vi "Start Measurement.vi"(8 "error in (no error)":errorcluster, 9 "Device Names":string[](array[string]), 10 "Measurement Name":string, 11 "Mag Lab Measure Controller in":refnum<class "Mag Lab Measure Controller.lvclass">) -> (0 "error out":errorcluster, 3 "Mag Lab Measure Controller out":refnum<class "Mag Lab Measure Controller.lvclass">)   [LabVIEW 2015, in "Mag Lab Measure Controller.lvclass"]
uses:
  Mag Lab Measure Controller.lvclass
  Mag Lab Root/Mag Lab Root.lvclass/Mag Lab Root.ctl
  <vilib>/ActorFramework/Actor/Actor.lvclass/Actor.ctl
  <vilib>/ActorFramework/Message Enqueuer/Message Enqueuer.lvclass/Message Enqueuer.ctl
  Mag Lab Measure Controller Messages/Log Status Update Msg/Log Status Update Msg.lvclass/Log Status Update Msg.ctl
  Mag Lab Root Messages/Initialize Msg/Initialize Msg.lvclass/Initialize Msg.ctl
  <vilib>/ActorFramework/Message Enqueuer/Init from Existing Queue.vi
  <vilib>/ActorFramework/Message Enqueuer/Enqueue.vi
  <vilib>/ActorFramework/Message Priority Queue/Priority Enqueue.vi
  <vilib>/ActorFramework/Message Enqueuer/Message Enqueuer.lvclass
  Mag Lab Measure Controller Messages/Log Status Update Msg/Log Status Update Msg.lvclass
  Mag Lab Root Messages/Initialize Msg/Initialize Msg.lvclass
  <vilib>/ActorFramework/Actor/Actor.lvclass
  Mag Lab Error Handler/Mag Lab Error Handler.lvclass
  Mag Lab Measure Base/Mag Lab Measure Base.lvclass
  Mag Lab Root/Mag Lab Root.lvclass
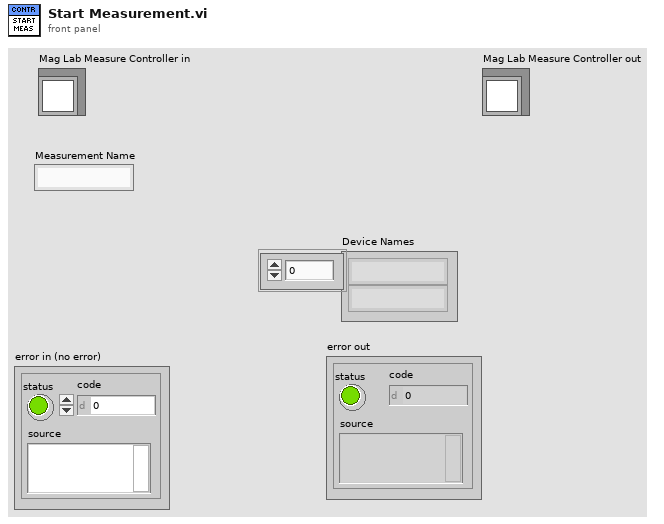
[diagram p1: front panel]
types:
  T1 = cluster{"Measurement Name":string, "Device Names":string[]}
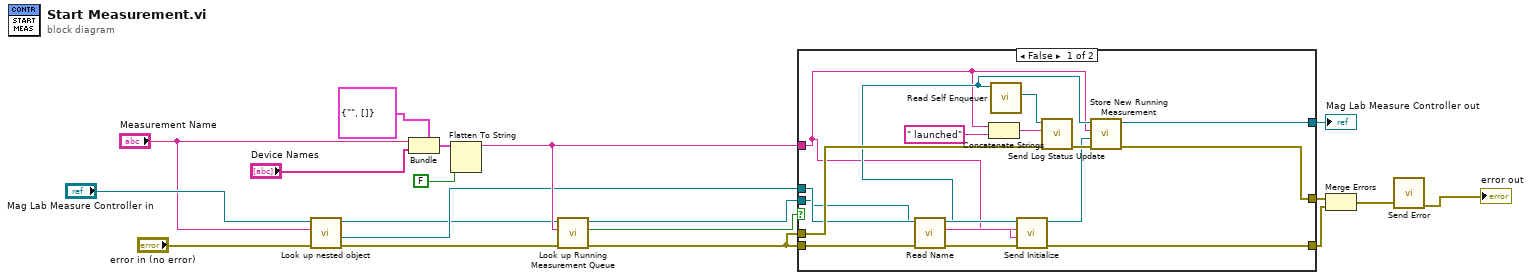
[diagram p0: block diagram]
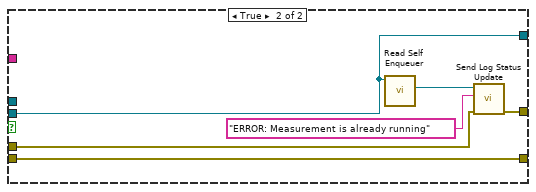
[diagram p2: hidden frame]
diagram:
  n1 = call "Look up nested object.vi"("error in (no error)"="error in (no error)", "Object name"="Measurement Name", "Mag Lab Measure Base in"="Mag Lab Measure Controller in") -> ("error out"=w2:errorcluster, "Object Queue"=w6:refnum<class "Message Enqueuer.lvclass">, "Mag Lab Measure Base out"=w5:refnum<class "Mag Lab Measure Controller.lvclass">)  [unwired: 5 in, 1 out]
  n2 = Bundle(cluster=T1 {"Measurement Name"="", "Device Names"=[]} ("output cluster"), "Measurement Name"="Measurement Name", "Device Names"="Device Names") -> (w18:T1)
  n3 = Flatten To String(anything=w18, prepend array or string size? (T)=FALSE) -> (data string=w14:string)  [unwired: 2 in, 2 out]
  n4 = call "Look up Running Measurement Queue .vi"("error in (no error)"=w2, "Measurement Name.Harware()"=w14, "Mag Lab Measure Controller in"=w5) -> ("error out"=w11:errorcluster, "Found?"=w13:bool, "Mag Lab Measure Controller out"=w12:refnum<class "Mag Lab Measure Controller.lvclass">)  [unwired: 4 in, 1 out]
  n5 = case shown="False" w13 {
    tunnel: [w35 w41] -> w10
    tunnel: w6 -> [w28 _]
    tunnel: w14 -> [w20 _]
    tunnel: w12 -> [w25 w41]
    tunnel: w11 -> [w30 w39]
    tunnel: [w33 w38] -> w15
    tunnel: w11 -> [w22 w40]
    tunnel: [w26 w40] -> w16
    frame False {
      n6 = call "Read Name.vi"("error in (no error)"=w22, "Mag Lab Root in"=w25) -> ("error out"=w23:errorcluster, "Name"=w21:string, "Mag Lab Root out"=w24:refnum<class "Mag Lab Measure Controller.lvclass">)  [unwired: 7 in]
      n7 = Concatenate Strings(w20, " launched" ("string")) -> (w31:string)
      n8 = call <vilib>:"Read Self Enqueuer.vi"("Actor"=w24) -> ("Self Enqueuer"=w32:refnum<class "Message Enqueuer.lvclass">)  [unwired: 10 in]
      n9 = call "Send Initialize.vi"("error in (no error)"=w23, "Requestor"=w21, "Requestee"=w20, "Message Enqueuer"=w28) -> ("error out"=w26:errorcluster, "Message Enqueuer out"=w27:refnum<class "Message Enqueuer.lvclass">)  [unwired: 6 in]
      n10 = call "Send Log Status Update.vi"("error in (no error)"=w30, "Status"=w31, "Message Enqueuer"=w32) -> ("error out"=w29:errorcluster)  [unwired: 7 in, 1 out]
      n11 = call "Store New Running Measurement.vi"("error in (no error)"=w29, "Caller-To-Actor Enqueuer"=w27, "name"=w20, "Mag Lab Measure Controller in"=w24) -> ("error out"=w33:errorcluster, "Mag Lab Measure Controller out"=w35:refnum<class "Mag Lab Measure Controller.lvclass">)  [unwired: 6 in]
    }
    frame True {
      n12 = call <vilib>:"Read Self Enqueuer.vi"("Actor"=w41) -> ("Self Enqueuer"=w37:refnum<class "Message Enqueuer.lvclass">)  [unwired: 10 in]
      n13 = call "Send Log Status Update.vi"("error in (no error)"=w39, "Status"="ERROR: Measurement is already running", "Message Enqueuer"=w37) -> ("error out"=w38:errorcluster)  [unwired: 7 in, 1 out]
    }
  }
  "Mag Lab Measure Controller out" <- w10
  n14 = Merge Errors(w15, w16) -> (w9:errorcluster)
  n15 = call "Send Error.vi"("error in (no error)"=w9) -> ("error out"=→"error out":errorcluster)  [unwired: 9 in, 1 out]
